vi "BuildMenu.vi"(0 "XRef":T8, 1 "MenuRef":T7, 2 "Point":T5, 3 "Menu Type":T4, 4 "State In":T2) -> (14 "Fatal Error Out":T1)   [LabVIEW 2018, in "RetryNode.xnode"]
uses:
  RetryNode.xnode
  <vilib>/XNodeSupport/XNodeXNodeRef.ctl
  <vilib>/XNodeSupport/XNodeMenuRef.ctl
  <vilib>/XNodeSupport/XNodePoint.ctl
  <vilib>/XNodeSupport/XNodeInt.ctl
  <vilib>/XNodeSupport/XNodeMenuType.ctl
  State.ctl
  <vilib>/Utility/miscctls.llb/LVRectTypeDef.ctl
  <vilib>/XNodeSupport/XNodeErrorCluster.ctl
  <vilib>/XNodeSupport/NI_XNodeSupport.lvlib
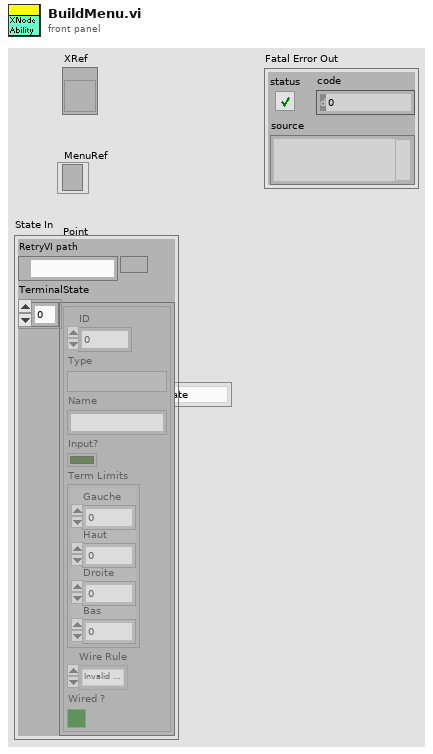
[diagram p1: front panel]
types:
  T1 = typedef "NI_XNodeSupport.lvlib/XNodeErrorCluster.ctl" = errorcluster
  T2 = typedef "RetryNode.xnode/State.ctl" = cluster{"RetryVI path":path, "TerminalState":cluster{"ID":i32, "Type":variant, "Name":string, "Input?":bool, "Term Limits":T3, "Wire Rule":enum16{"Invalid Wire Rule", "Required", "Recommended", "Optional", "Dynamic Dispatch"}, "Wired ?":bool}[]}
  T3 = typedef "LVRectTypeDef.ctl" = cluster{"Left":i16, "Top":i16, "Right":i16, "Bottom":i16}
  T4 = typedef "NI_XNodeSupport.lvlib/XNodeMenuType.ctl" = enum32{"Single Object Operate", "Single Object Popup", "Multi Object Popup Master", "Multi Object Popup Other"}
  T5 = typedef "NI_XNodeSupport.lvlib/XNodePoint.ctl" = cluster{"H":T6, "V":T6}
  T6 = typedef "NI_XNodeSupport.lvlib/XNodeInt.ctl" = i32
  T7 = typedef "NI_XNodeSupport.lvlib/XNodeMenuRef.ctl" = refnum<k9>
  T8 = typedef "NI_XNodeSupport.lvlib/XNodeXNodeRef.ctl" = refnum<vi>
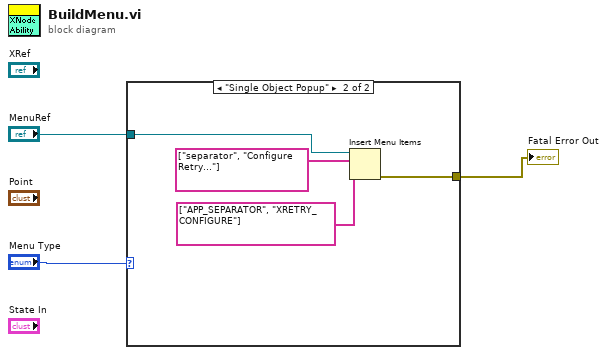
[diagram p0: block diagram]
diagram:
  n1 = case shown="\"Single Object Popup\"" "Menu Type" {
    tunnel: "MenuRef" -> [_ w7]
    tunnel: [_ w4] -> w1
    frame "Single Object Operate", Default {
    }
    frame "Single Object Popup" {
      n2 = Insert Menu Items(7:string[] ["APP_SEPARATOR", "XRETRY_CONFIGURE"] ("item tags"), 8:string[] ["separator", "Configure Retry..."] ("item names"), 9:w7) -> (0:w4:errorcluster)  [unwired: 3 in, 2 out]
    }
  }
  "Fatal Error Out" <- w1
